vi "ryerror_add_timestamp.vi"(2 "error in (no error)":errorcluster) -> (7 "error out":errorcluster)   [LabVIEW 2017]
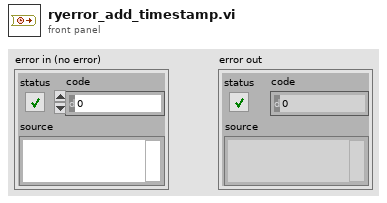
[diagram p1: front panel]
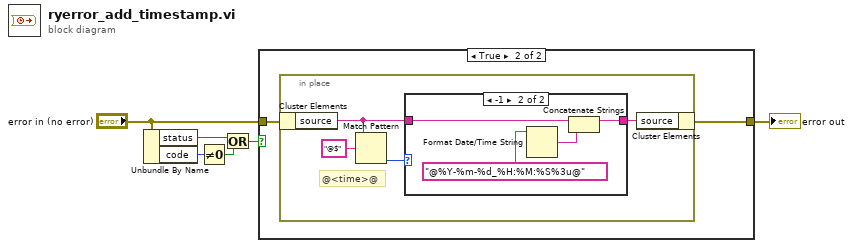
[diagram p0: block diagram]
diagram:
  n1 = Unbundle By Name("error in (no error)") -> ("status"=w5:bool, "code"=w4:i32)
  n2 = Not Equal To 0?(x=w4) -> (x != 0?=w3:bool)
  n3 = Or(x=w5, y=w3) -> (x .or. y?=w2:bool)
  n4 = case shown="True" w2 {
    tunnel: "error in (no error)" -> [w7 w9]
    tunnel: [w7 w8] -> w1
    frame False {
    }
    frame True {
      n5 = in-place {
        # "@<time>@"
        n6 = in-place-cluster #1(w9) -> ("source"=w12:string)
        n7 = Match Pattern(string=w12, regular expression="@$") -> (offset past match=w10:i32)  [unwired: 1 in, 3 out]
        n8 = case shown="-1" w10 {
          tunnel: w12 -> [w14 w18]
          tunnel: [w14 w17] -> w13
          frame Default {
          }
          frame -1 {
            n9 = Format Date/Time String(time format string (%c)="@%Y-%m-%d_%H:%M:%S%3u@") -> (date/time string=w16:string)  [unwired: 2 in]
            n10 = Concatenate Strings(w18, w16) -> (w17:string)
          }
        }
        n11 = in-place-cluster #1("source"=w13) -> (w8:errorcluster)
      }
    }
  }
  "error out" <- w1
